vi "Initialize Front Panel.vi"(8 "error in (no error)":errorcluster, 11 "For Loop Dialog in":refnum<class "TestStep Edit Dialog.lvclass">) -> (0 "error out":errorcluster, 3 "For Loop Dialog out":refnum<class "TestStep Edit Dialog.lvclass">)   [LabVIEW 2017, in "TestStep Edit Dialog.lvclass"]
doc: "<License>\nCopyright © 2017 Composed Systems, LLC | All rights reserved\nwww.composed.io\n\nAuthor: Ethan Stern <ethan.stern@composed.io>\n\nThis software is provided \"AS IS\" WITHOUT WARRANTIES, either express or implied, AND IS FOR EDUCATIONAL PURPOSES ONLY.\n</License>"
uses:
  <vilib>/gpm_packages/@cs/Test-executive-builder/Source/Test Executive Builder Dialogs/TestStep Edit Dialog/TestStep Edit Dialog.lvclass
  C:/Program Files/National Instruments/LabVIEW 2017/vi.lib/gpm_packages/@cs/popup-viewmanager/Source/Popup ViewManager/Popup ViewManager.lvclass
  <vilib>/gpm_packages/@cs/Test-executive-builder/Source/Test Executive Builder Dialogs/TestStep Edit Dialog/TestStep Edit Dialog.lvclass/TestStep Edit Dialog.ctl
  <vilib>/gpm_packages/@cs/mva-viewable/Source/IViewable/IViewable Messages/Insert Front Panel Msg/Insert Front Panel Msg.lvclass/Insert Front Panel Msg.ctl
  <vilib>/ActorFramework/Message Enqueuer/Message Enqueuer.lvclass/Message Enqueuer.ctl
  <vilib>/gpm_packages/@cs/Test-executive-builder/Source/Test Executive Builder Dialogs/IAttribute Data Type View Messages/Set Value Msg/Set Value Msg.lvclass/Set Value Msg.ctl
  <vilib>/ActorFramework/Message Enqueuer/Enqueue.vi
  <vilib>/gpm_packages/@cs/mva-viewable/Source/IViewable/IViewable Messages/Insert Front Panel Msg/Insert Front Panel Msg.lvclass
  C:/Program Files/National Instruments/LabVIEW 2017/vi.lib/ActorFramework/Message/Message.lvclass
  <vilib>/gpm_packages/@cs/Test-executive-builder/Source/Test Executive Builder Dialogs/IAttribute Data Type View Messages/Set Value Msg/Set Value Msg.lvclass
  <vilib>/ActorFramework/Message Priority Queue/Priority Enqueue.vi
  <vilib>/gpm_packages/@cs/Test-executive-builder/Source/Test Executive Builder Dialogs/ITest Executive Builder Dialog/ITest Executive Builder Dialog.lvclass
  <vilib>/gpm_packages/@cs/popup-viewmanager/Source/Popup ViewManager/Popup ViewManager.lvclass
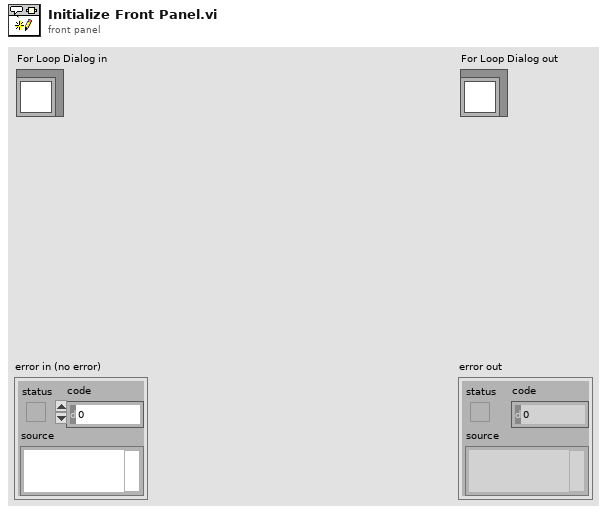
[diagram p1: front panel]
types:
  T1 = typedef "IViewable.lvlib/ProtectedSubpanel.lvclass/Protected Subpanel Reference.ctl" = refnum<data-value>
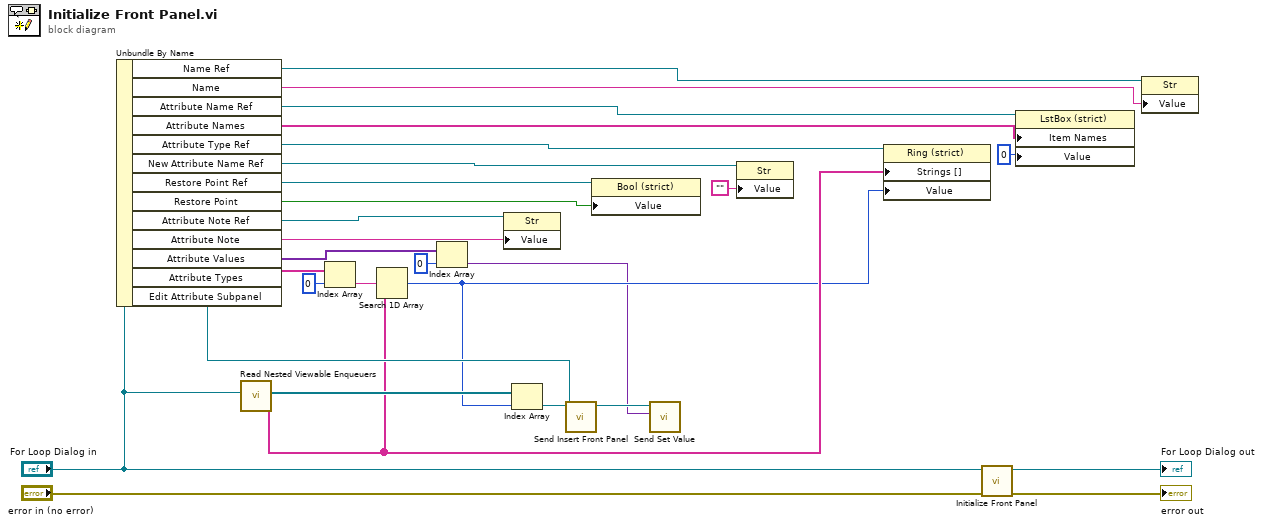
[diagram p0: block diagram]
diagram:
  n1 = Unbundle By Name("For Loop Dialog in") -> ("Name Ref"=w26:refnum<vi>, "Name"=w25:string, "Attribute Name Ref"=w23:refnum<vi>, "Attribute Names"=w22:string[], "Attribute Type Ref"=w20:refnum<vi>, "New Attribute Name Ref"=w19:refnum<vi>, "Restore Point Ref"=w17:refnum<vi>, "Restore Point"=w16:bool, "Attribute Note Ref"=w15:refnum<vi>, "Attribute Note"=w14:string, "Attribute Values"=w3:variant[], "Attribute Types"=w9:string[], "Edit Attribute Subpanel"=w10:T1)
  n2 = call <vilib>:"Read Nested Viewable Enqueuers.vi"("Popup ViewManager in"="For Loop Dialog in") -> ("Viewable Names"=w8:string[], "Nested Enqueuers"=w12:refnum<class "Message Enqueuer.lvclass">[])  [unwired: 9 in]
  n3 = Index Array(array=w9, index=0) -> (element=w7:string)
  n4 = Search 1D Array(1D array=w8, element=w7) -> (index of element=w5:i32)  [unwired: 1 in]
  n5 = Index Array(array=w3, index=0) -> (element=w1:variant)
  n6 = property class="Str"(reference=w15, "Value"=w14) -> ()  [unwired: 1 in, 2 out]
  n7 = Index Array(array=w12, index=w5) -> (element=w11:refnum<class "Message Enqueuer.lvclass">)
  n8 = call <vilib>:"Send Insert Front Panel.vi"("Protected Subpanel"=w10, "Message Enqueuer"=w11) -> ("Message Enqueuer out"=w2:refnum<class "Message Enqueuer.lvclass">)  [unwired: 8 in, 1 out]
  n9 = property class="Bool (strict)"(reference=w17, "Value"=w16) -> ()  [unwired: 1 in, 2 out]
  n10 = call <vilib>:"Send Set Value.vi"("Value"=w1, "Message Enqueuer"=w2) -> ()  [unwired: 8 in, 2 out]
  n11 = property class="Str"(reference=w19, "Value"="") -> ()  [unwired: 1 in, 2 out]
  n12 = property class="Ring (strict)"(reference=w20, "Strings []"=w8, "Value"=w5) -> ()  [unwired: 1 in, 2 out]
  n13 = call-parent "Initialize Front Panel.vi"("error in (no error)"="error in (no error)", "ITest Executive Builder Dialog in"="For Loop Dialog in") -> ("error out"=→"error out":errorcluster, "ITest Executive Builder Dialog out"=→"For Loop Dialog out":refnum<class "TestStep Edit Dialog.lvclass">)  [unwired: 8 in]
  n14 = property class="LstBox (strict)"(reference=w23, "Item Names"=w22, "Value"=u16 0) -> ()  [unwired: 1 in, 2 out]
  n15 = property class="Str"(reference=w26, "Value"=w25) -> ()  [unwired: 1 in, 2 out]
